vi "全局变量.vi"() -> ()   [LabVIEW 2018]
panel:
  out "排气量":dbl
  out "进空气量":dbl
  out "进蒸汽量":dbl
  out "1M8仓压力仿真":dbl
  out "1M8仓温度仿真":dbl
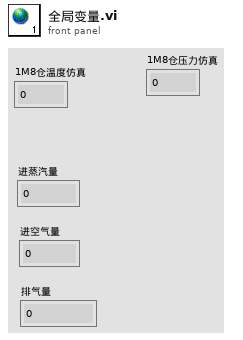
[diagram p1: front panel]
diagram:
